vi "Enqueue Message.vi"(8 "error in (no error)":errorcluster, 9 "Message Priority (Normal)":T1=enum."Normal", 10 "Message":refnum<class "Message.lvclass">, 11 "Interlock Q Class in":refnum<class "Interlock Q Class.lvclass">) -> (0 "error out":errorcluster, 3 "Interlock Q Class out":refnum<class "Interlock Q Class.lvclass">)   [LabVIEW 2022 SP3, in "Interlock Q Class.lvclass"]
uses:
  Interlock Q Class.lvclass
  Interlock Q Class.lvclass/Interlock Q Class.ctl
  <vilib>/ActorFramework/Message Enqueuer/Message Enqueuer.lvclass
  <vilib>/ErrorRing/Error Ring.xnode
  <vilib>/Utility/error.llb/Error Cluster From Error Code.vi
  Process State Data/Process State Data.lvclass
  <vilib>/ActorFramework/Message Enqueuer/Message Priority.ctl
  <vilib>/ActorFramework/Message/Message.lvclass
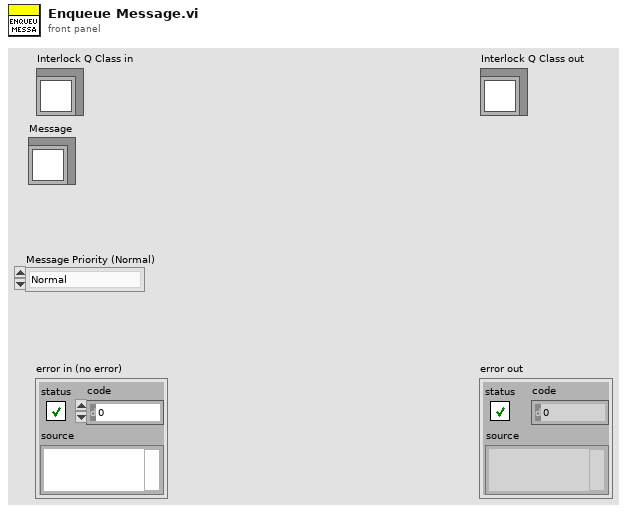
[diagram p1: front panel]
types:
  T1 = typedef "Actor Framework.lvlib/Message Enqueuer.lvclass/Message Priority.ctl" = enum16{"Low", "Normal", "High"}
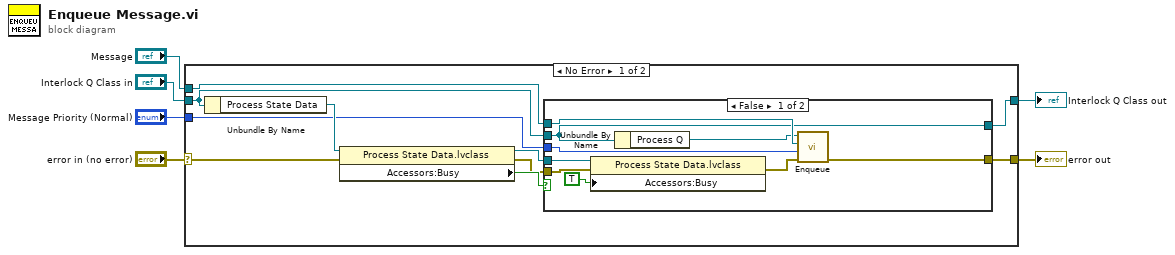
[diagram p0: block diagram]
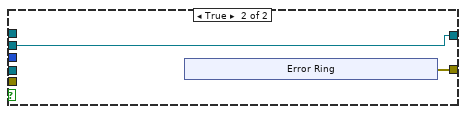
[diagram p2: hidden frame]
diagram:
  n1 = case shown="No Error" "error in (no error)" {
    selector: "error in (no error)" -> [w9 w34]
    tunnel: [w13 w34] -> w5
    tunnel: [w7 w33] -> w3
    tunnel: "Interlock Q Class in" -> [w8 w33]
    tunnel: "Message" -> [w15 _]
    tunnel: "Message Priority (Normal)" -> [w14 _]
    frame No Error {
      n2 = Unbundle By Name(w8) -> ("Process State Data"=w16:refnum<data-value>)
      n3 = property class="Process State Data.lvclass"(reference=w16, error in=w9) -> (reference out=w11:refnum<data-value>, error out=w10:errorcluster, "Accessors:Busy"=w12:bool)
      n4 = case shown="False" w12 {
        tunnel: w15 -> [w25 _]
        tunnel: w14 -> [w24 _]
        tunnel: [w23 w27] -> w13
        tunnel: w11 -> [w22 _]
        tunnel: w10 -> [w20 _]
        tunnel: w8 -> [w17 w26]
        tunnel: [w17 w26] -> w7
        frame False {
          n5 = property class="Process State Data.lvclass"(reference=w22, error in=w20, "Accessors:Busy"=TRUE ("Busy")) -> (error out=w19:errorcluster)  [unwired: 1 out]
          n6 = Unbundle By Name(w17) -> ("Process Q"=w18:refnum<class "Message Enqueuer.lvclass">)
          n7 = call <vilib>:"Enqueue.vi"("error in (no error)"=w19, "Message Priority (Normal)"=w24, "Message"=w25, "Message Enqueuer in"=w18) -> ("error out"=w23:errorcluster)  [unwired: 6 in, 1 out]
        }
        frame True {
          n8 = xnode "Error Ring"() -> ("error out"=w27:errorcluster)
        }
      }
    }
    frame Error {
    }
  }
  "error out" <- w5
  "Interlock Q Class out" <- w3
